vi "Assert Update UserInfo.vi"() -> ()   [LabVIEW 2015, in "Information.lvclass"]
uses:
  Information.lvclass
  Type Definitions/UserInfo.ctl
  Information.lvclass/Information.ctl
panel:
  out "UserInfo 2":T1
  in  "Boolean":bool
  in  "UserInfo":T1
  in  "组别":enum16{"电控", "机械", "视觉"}(ring)
  in  "部门":string
  in  "操作资料":bool caption="修改信息"
  in  "点击上传照片":bool
  in  "学院":string
  in  "QQ":string
  in  "电话":string
  in  "邮箱":string
  in  "性别":enum16{"男", "女"}(ring)
  out "照片":picture
  in  "学号":string
  in  "年龄":dbl
  in  "姓名":string
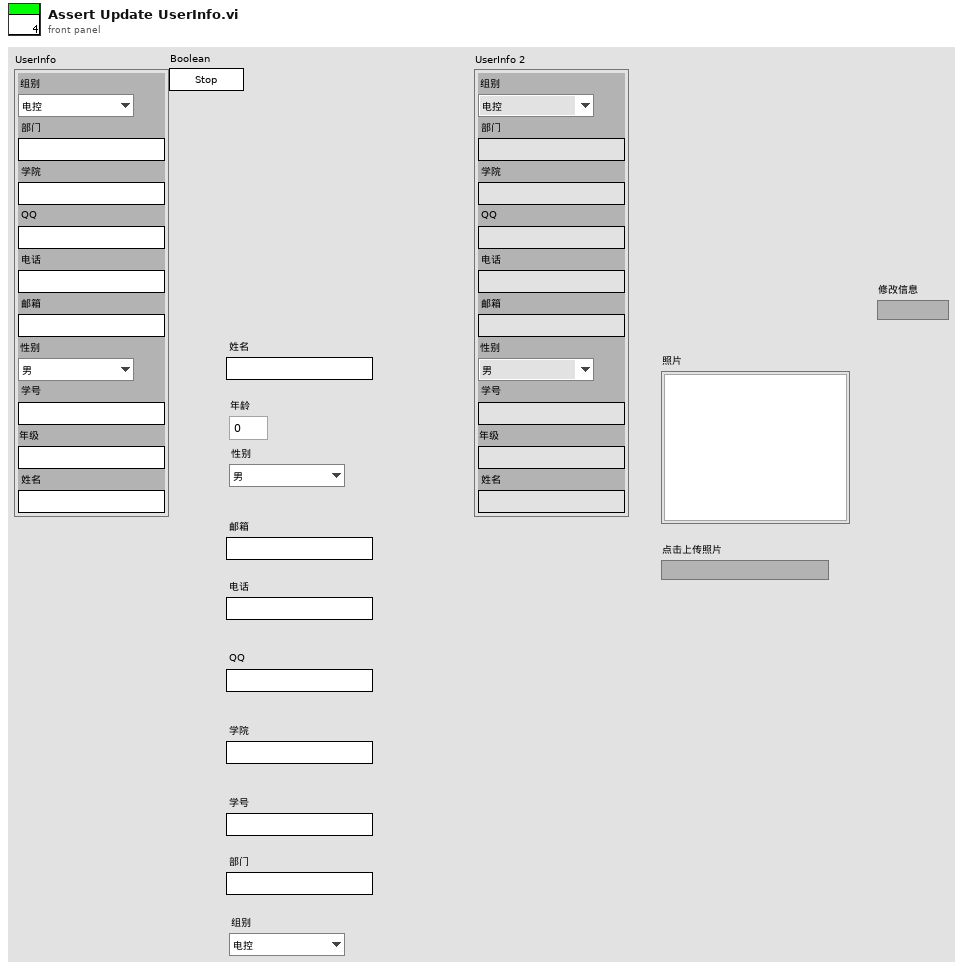
[diagram p1: front panel]
types:
  T1 = typedef "Information.lvclass/UserInfo.ctl" = cluster{"组别":enum16{"电控", "机械", "视觉"}, "部门":string, "学院":string, "QQ":string, "电话":string, "邮箱":string, "性别":enum16{"男", "女"}, "学号":string, "年级":string, "姓名":string}
  T2 = cluster{"姓名":refnum<vi>, "年龄":refnum<vi>, "学号":refnum<vi>, "照片":refnum<vi>, "性别":refnum<vi>, "邮箱":refnum<vi>, "电话":refnum<vi>, "QQ":refnum<vi>, "学院":refnum<vi>, "点击上传照片":refnum<vi>, "操作资料":refnum<vi>, "部门":refnum<vi>, "组别":refnum<vi>}
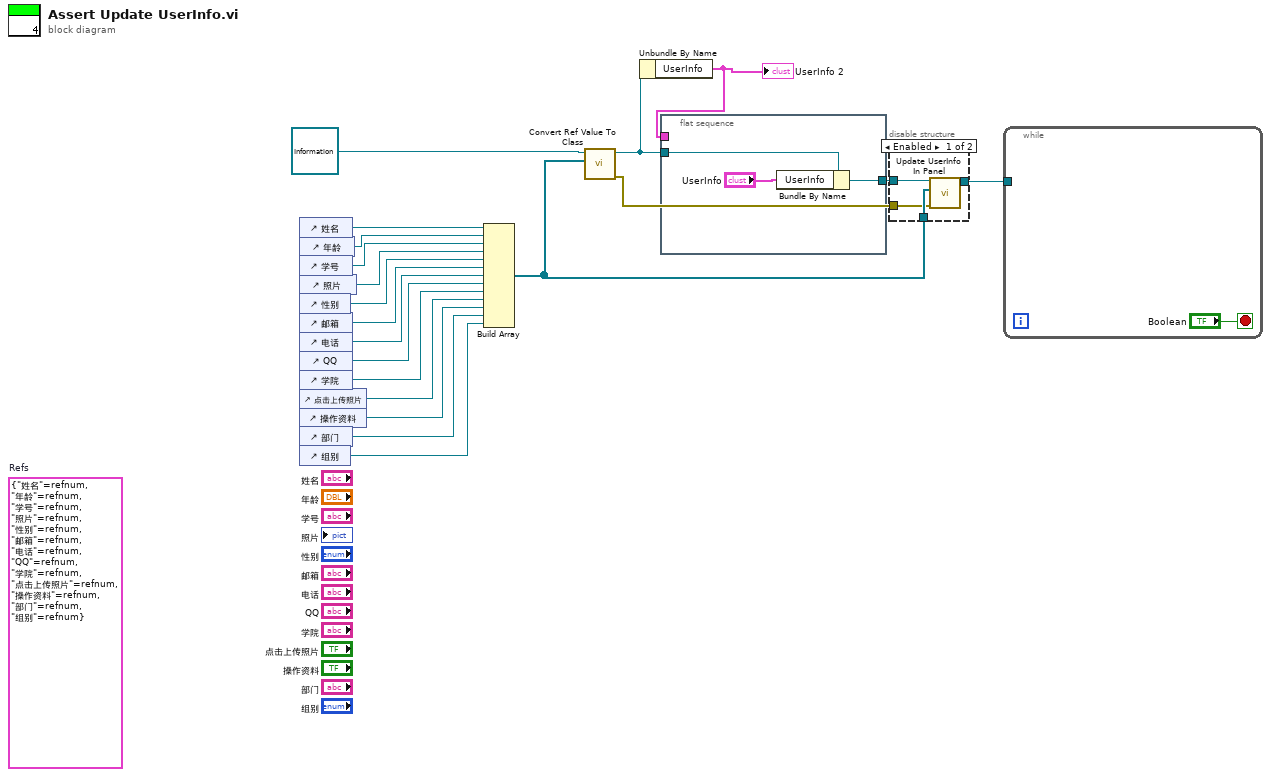
[diagram p0: block diagram]
diagram:
  (unwired) T2 {"姓名"=refnum, "年龄"=refnum, "学号"=refnum, "照片"=refnum, "性别"=refnum, "邮箱"=refnum, "电话"=refnum, "QQ"=refnum, "学院"=refnum, "点击上传照片"=refnum, "操作资料"=refnum, "部门"=refnum, "组别"=refnum}  # Refs
  n1 = control-ref of="姓名"() -> (w18:refnum<vi>)
  n2 = control-ref of="年龄"() -> (w17:refnum<vi>)
  n3 = control-ref of="学号"() -> (w16:refnum<vi>)
  n4 = control-ref of="照片"() -> (w15:refnum<vi>)
  n5 = control-ref of="性别"() -> (w14:refnum<vi>)
  n6 = control-ref of="邮箱"() -> (w13:refnum<vi>)
  n7 = control-ref of="电话"() -> (w12:refnum<vi>)
  n8 = control-ref of="QQ"() -> (w11:refnum<vi>)
  n9 = control-ref of="学院"() -> (w10:refnum<vi>)
  n10 = control-ref of="点击上传照片"() -> (w9:refnum<vi>)
  n11 = control-ref of="操作资料"() -> (w8:refnum<vi>)
  n12 = control-ref of="部门"() -> (w7:refnum<vi>)
  n13 = control-ref of="组别"() -> (w6:refnum<vi>)
  n14 = Build Array(w18, w17, w16, w15, w14, w13, w12, w11, w10, w9, w8, w7, w6) -> (w4:refnum<vi>[])
  n15 = call "Convert Ref Value To Class.vi"("Main Ctls and VI Refs"=w4, "MemberInfo in"=refnum<class "Information.lvclass"> refnum ("Member_Actor.lvlib:MemberInfo.lvclass")) -> ("error out"=w3:errorcluster, "MemberInfo out"=w2:refnum<class "Information.lvclass">)  [unwired: 8 in]
  n16 = Unbundle By Name(w2) -> ("UserInfo"=w1:T1)
  "UserInfo 2" <- w1
  n17 = flat-sequence {
    tunnel: [w23] -> w20
    tunnel: w2 -> [w21]
    tunnel: w1 -> [_]
    frame #0 {
      n18 = Bundle By Name(cluster=w21, "UserInfo"="UserInfo") -> (w23:refnum<class "Information.lvclass">)
    }
  }
  n19 = disable-structure shown="Enabled" {
    disable-tunnel: w20 -> [w27 _]
    disable-tunnel: [w26 _] -> w19
    disable-tunnel: w4 -> [w25 _]
    disable-tunnel: w3 -> [w24 _]
    frame Enabled {
      n20 = call "Update UserInfo In Panel.vi"("error in (no error)"=w24, "UI Ref"=w25, "MemberInfo in"=w27) -> ("MemberInfo out"=w26:refnum<class "Information.lvclass">)  [unwired: 6 in, 2 out]
    }
    frame Disabled {
    }
  }
  n21 = while {
    tunnel: w19 -> [_]
    stop <- "Boolean" stop-if-true
  }
